vi "Test Bench Constants Linux x64.vi"() -> (1 "Deployment Hooks class":refnum<class "Custom Device Deployment Hooks.lvclass">, 3 "Custom Device class":refnum<class "Custom Device.lvclass">)   [LabVIEW 2026]
uses:
  <userlib>/Custom Device Interfaces_v1.lvlibp/CustomDevice/Custom Device.lvclass
  <userlib>/Custom Device Interfaces_v1.lvlibp/CustomDeviceDeploymentHooks/Custom Device Deployment Hooks.lvclass
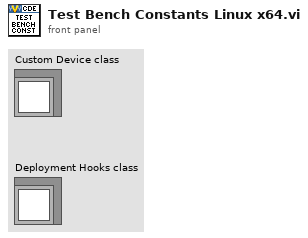
[diagram p1: front panel]
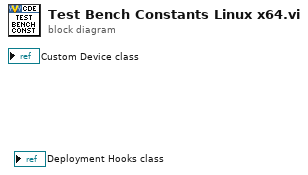
[diagram p0: block diagram]
diagram:
